vi "ConsumerPast.vi"(5 "Day of Year":u32, 6 "Unique Object Identifier":string, 7 "Day Time":u32, 8 "Error In":errorcluster, 10 "Energy flow IN":T2, 11 "DataFlowIN":T1) -> (0 "Error Out":errorcluster, 2 "Energy flow OUT":T2, 3 "DataFlowOUT":T1)   [LabVIEW 2017]
uses:
  classes/DataCollector.lvclass
  classes/DataHandler.lvclass
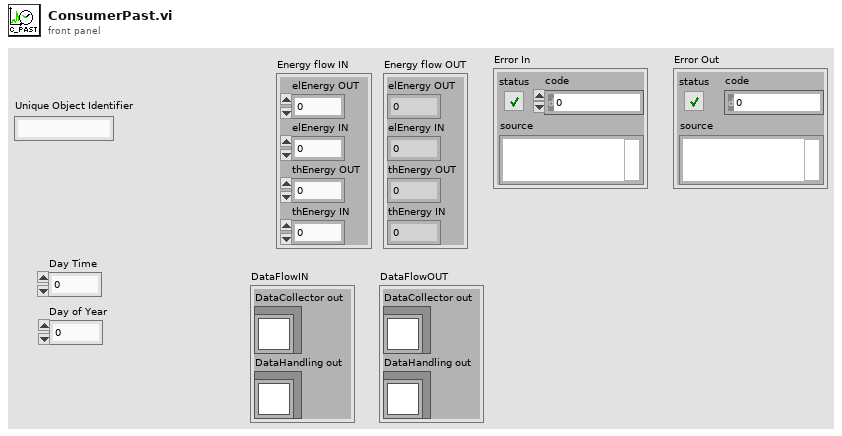
[diagram p1: front panel]
types:
  T1 = cluster{"DataCollector out":refnum<class "DataCollector.lvclass">, "DataHandling out":refnum<class "DataHandler.lvclass">}
  T2 = cluster{"elEnergy OUT":dbl, "elEnergy IN":dbl, "thEnergy OUT":dbl, "thEnergy IN":dbl}
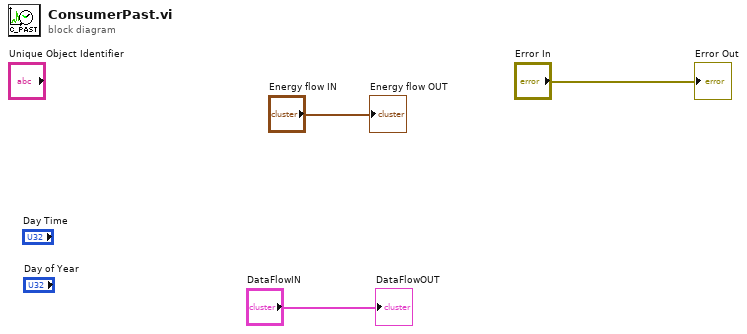
[diagram p0: block diagram]
diagram:
  "Error Out" <- "Error In"
  "Energy flow OUT" <- "Energy flow IN"
  "DataFlowOUT" <- "DataFlowIN"
